vi "Anritsu VNA Set Trace Display.vi"(4 "Trace":i8=1 min=1 max=99 step=1, 6 "Channel":i8=1 min=1 max=99 step=1, 7 "Anritsu VNA":T1, 8 "error in (no error)":errorcluster, 11 "VISA Resource Name":refnum<visa-resource-name>) -> (0 "error out":errorcluster, 3 "dup VISA Resource Name":refnum<visa-resource-name>)   [LabVIEW 2011]
uses:
  TypeDefs/Anritsu VNA Instrument Info.ctl
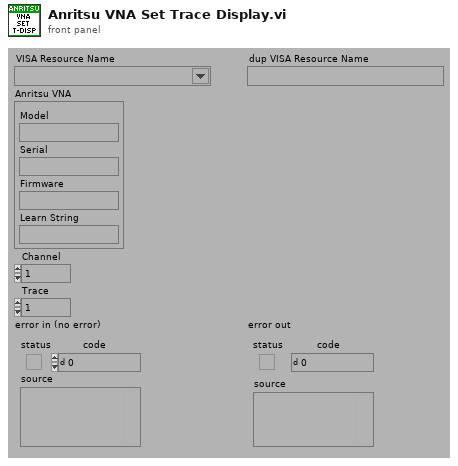
[diagram p1: front panel]
types:
  T1 = typedef "Anritsu VNA Instrument Info.ctl" = cluster{"Model":string, "Serial":string, "Firmware":string, "Learn String":string}
  T2 = typedef "Anritsu VNA Model.ctl" = enum16{"Not Supported", "37XXXX", "MS20XXX", "MS462XX", "MS464XX"}
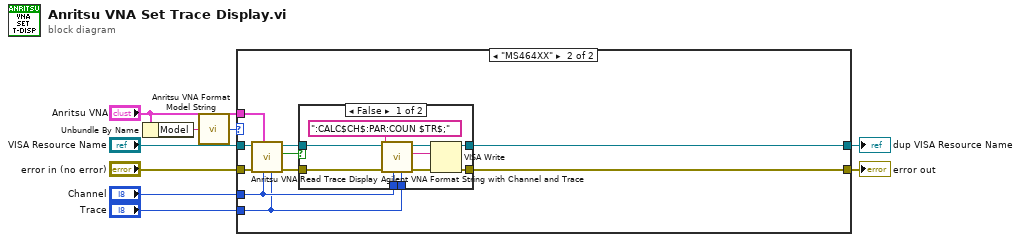
[diagram p0: block diagram]
diagram:
  n1 = Unbundle By Name("Anritsu VNA") -> ("Model"=w2:string)
  n2 = call "Anritsu VNA Format Model String.vi"("Model"=w2) -> ("Model"=w5:T2)
  n3 = case shown="\"MS464XX\"" w5 {
    tunnel: "VISA Resource Name" -> [w11 w18]
    tunnel: "error in (no error)" -> [w10 w19]
    tunnel: [w11 w21] -> w7
    tunnel: [w10 w20] -> w6
    tunnel: "Channel" -> [_ w14]
    tunnel: "Anritsu VNA" -> [_ w15]
    tunnel: "Trace" -> [_ w13]
    frame "Not Supported".."MS462XX" {
    }
    frame "MS464XX" {
      n4 = call "Anritsu VNA Read Trace Display.vi"("Trace"=w13, "Channel"=w14, "Anritsu VNA"=w15, "error in (no error)"=w19, "VISA Resource Name"=w18) -> ("error out"=w16:errorcluster, "Displayed?"=w12:bool, "dup VISA Resource Name"=w17:refnum<visa-resource-name>)  [unwired: 4 out]
      n5 = case shown="False" w12 {
        tunnel: [w29 w31] -> w21
        tunnel: [w28 w30] -> w20
        tunnel: w17 -> [w27 w31]
        tunnel: w16 -> [w26 w30]
        tunnel: w14 -> [w24 _]
        tunnel: w13 -> [w23 _]
        frame False {
          n6 = call "Agilent VNA Format String with Channel and Trace.vi"("Trace"=w23, "Channel"=w24, "String"=":CALC$CH$:PAR:COUN $TR$;" ("write buffer")) -> ("String Out"=w25:string)  [unwired: 6 out]
          n7 = VISA Write(VISA resource name=w27, write buffer=w25, error in (no error)=w26) -> (VISA resource name out=w29:refnum<visa-resource-name>, error out=w28:errorcluster)  [unwired: 1 out]
        }
        frame True {
        }
      }
    }
  }
  "dup VISA Resource Name" <- w7
  "error out" <- w6
